vi "FVI_Manette_Calcul Direction.vi"(9 "Axe L Y":dbl, 10 "Axe L X":dbl, 11 "Gain":dbl) -> (0 "Angle":dbl, 1 "Vitesse":dbl, 2 "Y":dbl, 3 "X":dbl)   [LabVIEW 2018]
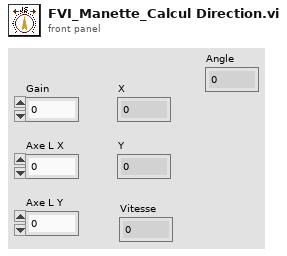
[diagram p1: front panel]
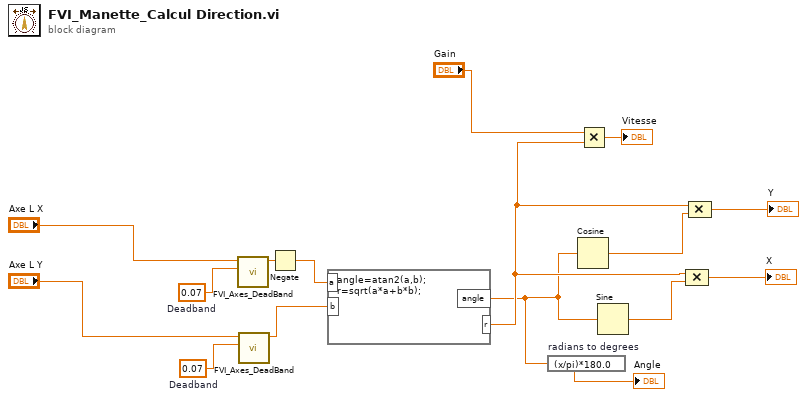
[diagram p0: block diagram]
diagram:
  w10 = 0.07  # Deadband
  w8 = 0.07  # Deadband
  n1 = call "FVI_Axes_DeadBand.vi"("deadband Value"=w8, "X axis in"="Axe L X") -> ("X axis out"=w9:dbl)  [unwired: 8 in, 1 out]
  n2 = call "FVI_Axes_DeadBand.vi"("deadband Value"=w10, "X axis in"="Axe L Y") -> ("X axis out"=w11:dbl)  [unwired: 8 in, 1 out]
  n3 = Negate(x=w9) -> (-x=w16:dbl)
  n4 = formula code="angle=atan2(a,b);\nr=sqrt(a*a+b*b);"("a"=w16, "b"=w11) -> ("angle"=w2:dbl, "r"=w5:dbl)
  n5 = expression code="(x/pi)*180.0" "radians to degrees"(w2) -> (→"Angle":dbl)
  n6 = Cosine(x=w2) -> (cos(x)=w12:dbl)
  n7 = Multiply(x="Gain", y=w5) -> (x*y=→"Vitesse":dbl)
  n8 = Sine(x=w2) -> (sin(x)=w13:dbl)
  n9 = Compound Arithmetic op=MULTIPLY(w5, w13) -> (→"X":dbl)
  n10 = Compound Arithmetic op=MULTIPLY(w5, w12) -> (→"Y":dbl)
